vi "set_rate.vi"(4 "error in (no error)":errorcluster, 5 "Set Rate":dbl, 7 "VISA resource name in":refnum<visa-resource-name>) -> (0 "error out":errorcluster, 3 "VISA resource name out":refnum<visa-resource-name>)   [LabVIEW 2017]
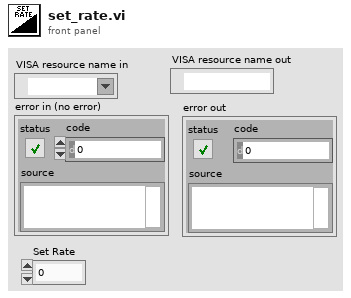
[diagram p1: front panel]
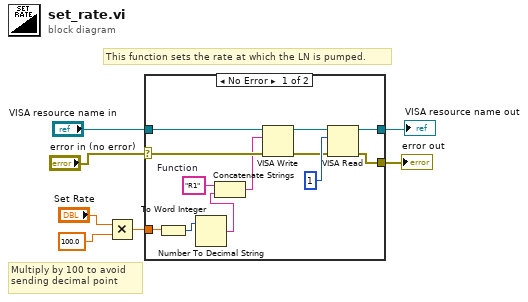
[diagram p0: block diagram]
diagram:
  # "This function sets the rate at which the LN is pumped."
  # "Multiply by 100 to avoid \nsending decimal point"
  n1 = Multiply(x="Set Rate", y=100.0) -> (x*y=w4:dbl)
  n2 = case shown="No Error" "error in (no error)" {
    selector: "error in (no error)" -> [w18 w20]
    tunnel: "VISA resource name in" -> [w19 w21]
    tunnel: w4 -> [w9 _]
    tunnel: [w11 w21] -> w3
    tunnel: [w10 w20] -> w2
    frame No Error {
      w17 = "R1"  # Function
      n3 = To Word Integer(number=w9) -> (16bit integer=w8:i16)
      n4 = Number To Decimal String(number=w8) -> (decimal integer string=w16:string)  [unwired: 1 in]
      n5 = Concatenate Strings(w17, w16) -> (w15:string)
      n6 = VISA Write(VISA resource name=w19, write buffer=w15, error in (no error)=w18) -> (VISA resource name out=w14:refnum<visa-resource-name>, error out=w12:errorcluster)  [unwired: 1 out]
      n7 = VISA Read(VISA resource name=w14, byte count=u32 1, error in (no error)=w12) -> (VISA resource name out=w11:refnum<visa-resource-name>, error out=w10:errorcluster)  [unwired: 2 out]
    }
    frame Error {
    }
  }
  "VISA resource name out" <- w3
  "error out" <- w2
